vi "ProfiledPIDController_Calculate_Meas.vi"(10 "PV-Measurement":dbl, 11 "in PROFILED_PID_CONTROLLER":T1={"Controller"={"Kp"=0.0, "Ki"=0.0, "Kd"=0.0, "Period"=0.0, "Max_Integral"=1.0, "Min_Integral"=-1.0, "Max_Input"=0.0, "Min_Input"=0.0, "Continuous"=FALSE, "PositionError"=0.0, "VelocityError"=0.0, "PrevError"=0.0, "TotalError"=0.0, "PositionTolerance"=0.05, "VelocityTolerance"=9.99e+35, "SetPoint"=0.0, "Kf"=0.0, "Prev_Deriv"=0.0, "Prev_Deriv 2"=0.0, "DerivativeFilter"=FALSE, "Min_Output"=-9.99e+35, "Max_Output"=9.9e+35, "Prev_F_P"=0.0, "Prev_F_P_2"=0.0, "AntiWindupActive"=FALSE, "Measurement"=0.0}, "Goal"={"Position"=0.0, "Velocity"=0.0}, "Setpoint"={"Position"=0.0, "Velocity"=0.0}, "Constraint"={"MaxVelocity"=0.0, "MaxAcceleration"=0.0}} {"Constraint"."MaxAcceleration" format="%16_6e"; "Constraint"."MaxVelocity" format="%16_6e"; "Setpoint"."Velocity" format="%16_6e"; "Setpoint"."Position" format="%16_6e"; "Goal"."Velocity" format="%16_6e"; "Goal"."Position" format="%16_6e"; "Controller"."Measurement" format="%16_6e"; "Controller"."Prev_F_P_2" format="%16_6e"; "Controller"."Prev_F_P" format="%16_6e"; "Controller"."Max_Output" format="%16_6e"; "Controller"."Min_Output" format="%16_6e"; "Controller"."Prev_Deriv 2" format="%16_6e"; "Controller"."Prev_Deriv" format="%16_6e"; "Controller"."Kf" format="%16_6e"; "Controller"."SetPoint" format="%16_6e"; "Controller"."VelocityTolerance" format="%16_6e"; "Controller"."PositionTolerance" format="%16_6e"; "Controller"."TotalError" format="%16_6e"; "Controller"."PrevError" format="%16_6e"; "Controller"."VelocityError" format="%16_6e"; "Controller"."PositionError" format="%16_6e"; "Controller"."Min_Input" format="%16_6e"; "Controller"."Max_Input" format="%16_6e"; "Controller"."Min_Integral" format="%16_6e"; "Controller"."Max_Integral" format="%16_6e"; "Controller"."Period" format="%16_6e"; "Controller"."Kd" format="%16_6e"; "Controller"."Ki" format="%16_6e"; "Controller"."Kp" format="%16_6e"}) -> (1 "CO-ControlOutput":dbl, 3 "out PROFILED_PID_CONTROLLER":T1={"Controller"={"Kp"=0.0, "Ki"=0.0, "Kd"=0.0, "Period"=0.0, "Max_Integral"=1.0, "Min_Integral"=-1.0, "Max_Input"=0.0, "Min_Input"=0.0, "Continuous"=FALSE, "PositionError"=0.0, "VelocityError"=0.0, "PrevError"=0.0, "TotalError"=0.0, "PositionTolerance"=0.05, "VelocityTolerance"=9.99e+35, "SetPoint"=0.0, "Kf"=0.0, "Prev_Deriv"=0.0, "Prev_Deriv 2"=0.0, "DerivativeFilter"=FALSE, "Min_Output"=-9.99e+35, "Max_Output"=9.9e+35, "Prev_F_P"=0.0, "Prev_F_P_2"=0.0, "AntiWindupActive"=FALSE, "Measurement"=0.0}, "Goal"={"Position"=0.0, "Velocity"=0.0}, "Setpoint"={"Position"=0.0, "Velocity"=0.0}, "Constraint"={"MaxVelocity"=0.0, "MaxAcceleration"=0.0}} {"Constraint"."MaxAcceleration" format="%16_6e"; "Constraint"."MaxVelocity" format="%16_6e"; "Setpoint"."Velocity" format="%16_6e"; "Setpoint"."Position" format="%16_6e"; "Goal"."Velocity" format="%16_6e"; "Goal"."Position" format="%16_6e"; "Controller"."Measurement" format="%16_6e"; "Controller"."Prev_F_P_2" format="%16_6e"; "Controller"."Prev_F_P" format="%16_6e"; "Controller"."Max_Output" format="%16_6e"; "Controller"."Min_Output" format="%16_6e"; "Controller"."Prev_Deriv 2" format="%16_6e"; "Controller"."Prev_Deriv" format="%16_6e"; "Controller"."Kf" format="%16_6e"; "Controller"."SetPoint" format="%16_6e"; "Controller"."VelocityTolerance" format="%16_6e"; "Controller"."PositionTolerance" format="%16_6e"; "Controller"."TotalError" format="%16_6e"; "Controller"."PrevError" format="%16_6e"; "Controller"."VelocityError" format="%16_6e"; "Controller"."PositionError" format="%16_6e"; "Controller"."Min_Input" format="%16_6e"; "Controller"."Max_Input" format="%16_6e"; "Controller"."Min_Integral" format="%16_6e"; "Controller"."Max_Integral" format="%16_6e"; "Controller"."Period" format="%16_6e"; "Controller"."Kd" format="%16_6e"; "Controller"."Ki" format="%16_6e"; "Controller"."Kp" format="%16_6e"})   [LabVIEW 2019, in "Trajectory_Library.lvlib"]
doc: "Returns the next output of the PID controller.\n\nInputs:\n - Profiled_PID_Controller -- Profiled_PID_Controller data cluster\n - measurement -- The current measurement of the process variable.\n\nOutputs:\n - Profiled_PID_Controller -- Updated Profiled_PID_Controller data cluster\n - CO-ControlOutput -- Calculated PID output"
uses:
  Trajectory_Library.lvlib
  PROFILED_PID_CONTROLLER.ctl
  PID_CONTROLLER.ctl
  TRAPEZOID_PROFILE_STATE.ctl
  TRAPEZOID_PROFILE_CONSTRAINT.ctl
  PIDController_SetSetpoint.vi
  PIDController_Calculate_PV.vi
  TrapProfile_ShouldFlipAcceleration.vi
  TrapProfile_Direct.vi
  <vilib>/Rock Robotics/SystemInterfaces/NetworkCommunication/NetComm_UsageReport_report.vi
  PIDController_GetPeriod.vi
  TrapProfState_New.vi
  Util_LibraryGlobals.vi
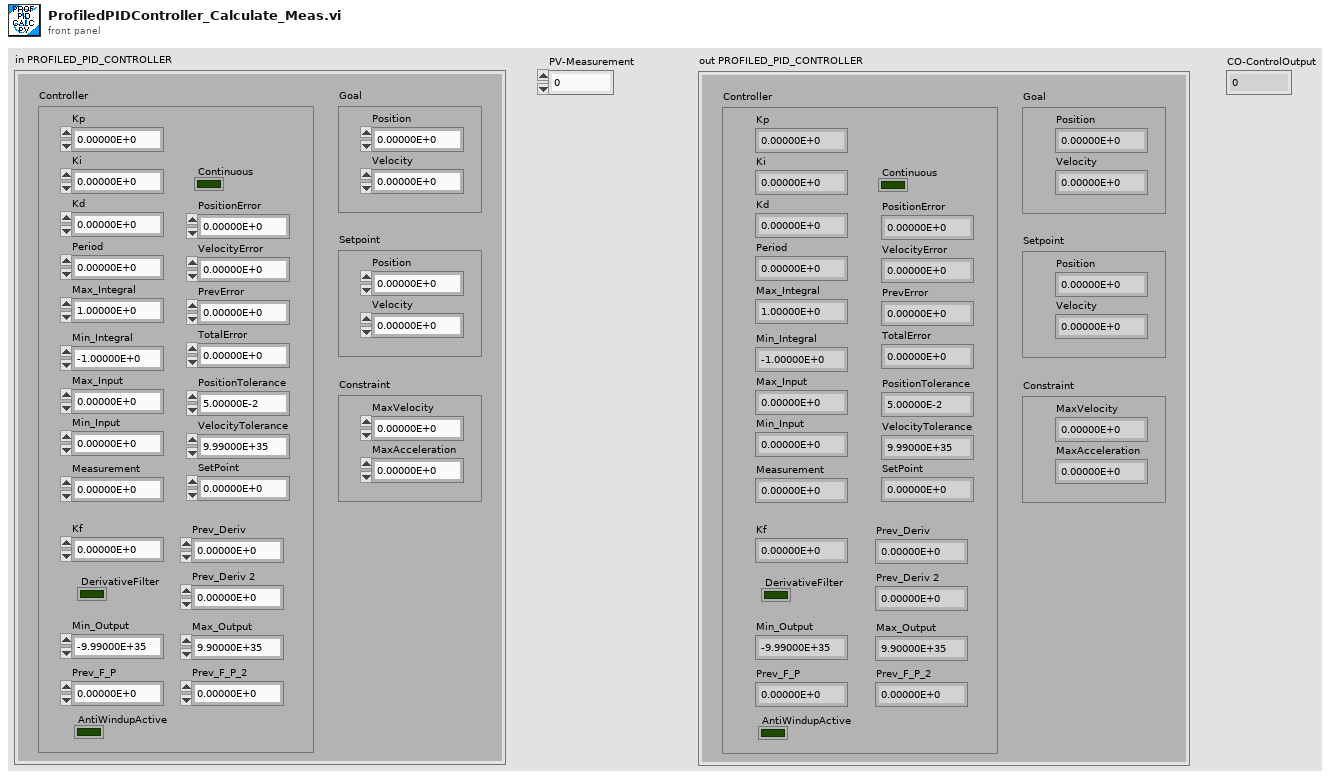
[diagram p1: front panel]
types:
  T1 = typedef "Trajectory_Library.lvlib/PROFILED_PID_CONTROLLER.ctl" = cluster{"Controller":T2, "Goal":T3, "Setpoint":T3, "Constraint":T4}
  T2 = typedef "Trajectory_Library.lvlib/PID_CONTROLLER.ctl" = cluster{"Kp":dbl, "Ki":dbl, "Kd":dbl, "Period":dbl, "Max_Integral":dbl, "Min_Integral":dbl, "Max_Input":dbl, "Min_Input":dbl, "Continuous":bool, "PositionError":dbl, "VelocityError":dbl, "PrevError":dbl, "TotalError":dbl, "PositionTolerance":dbl, "VelocityTolerance":dbl, "SetPoint":dbl, "Kf":dbl, "Prev_Deriv":dbl, "Prev_Deriv 2":dbl, "DerivativeFilter":bool, "Min_Output":dbl, "Max_Output":dbl, "Prev_F_P":dbl, "Prev_F_P_2":dbl, "AntiWindupActive":bool, "Measurement":dbl}
  T3 = typedef "Trajectory_Library.lvlib/TRAPEZOID_PROFILE_STATE.ctl" = cluster{"Position":dbl, "Velocity":dbl}
  T4 = typedef "Trajectory_Library.lvlib/TRAPEZOID_PROFILE_CONSTRAINT.ctl" = cluster{"MaxVelocity":dbl, "MaxAcceleration":dbl}
  T5 = typedef "Trajectory_Library.lvlib/TRAPEZOID_PROFILE.ctl" = cluster{"EndAccel":dbl, "EndFullSpeed":dbl, "EndDecel":dbl, "Direction":i32, "Constraints":T4, "Initial":T3, "Goal":T3}
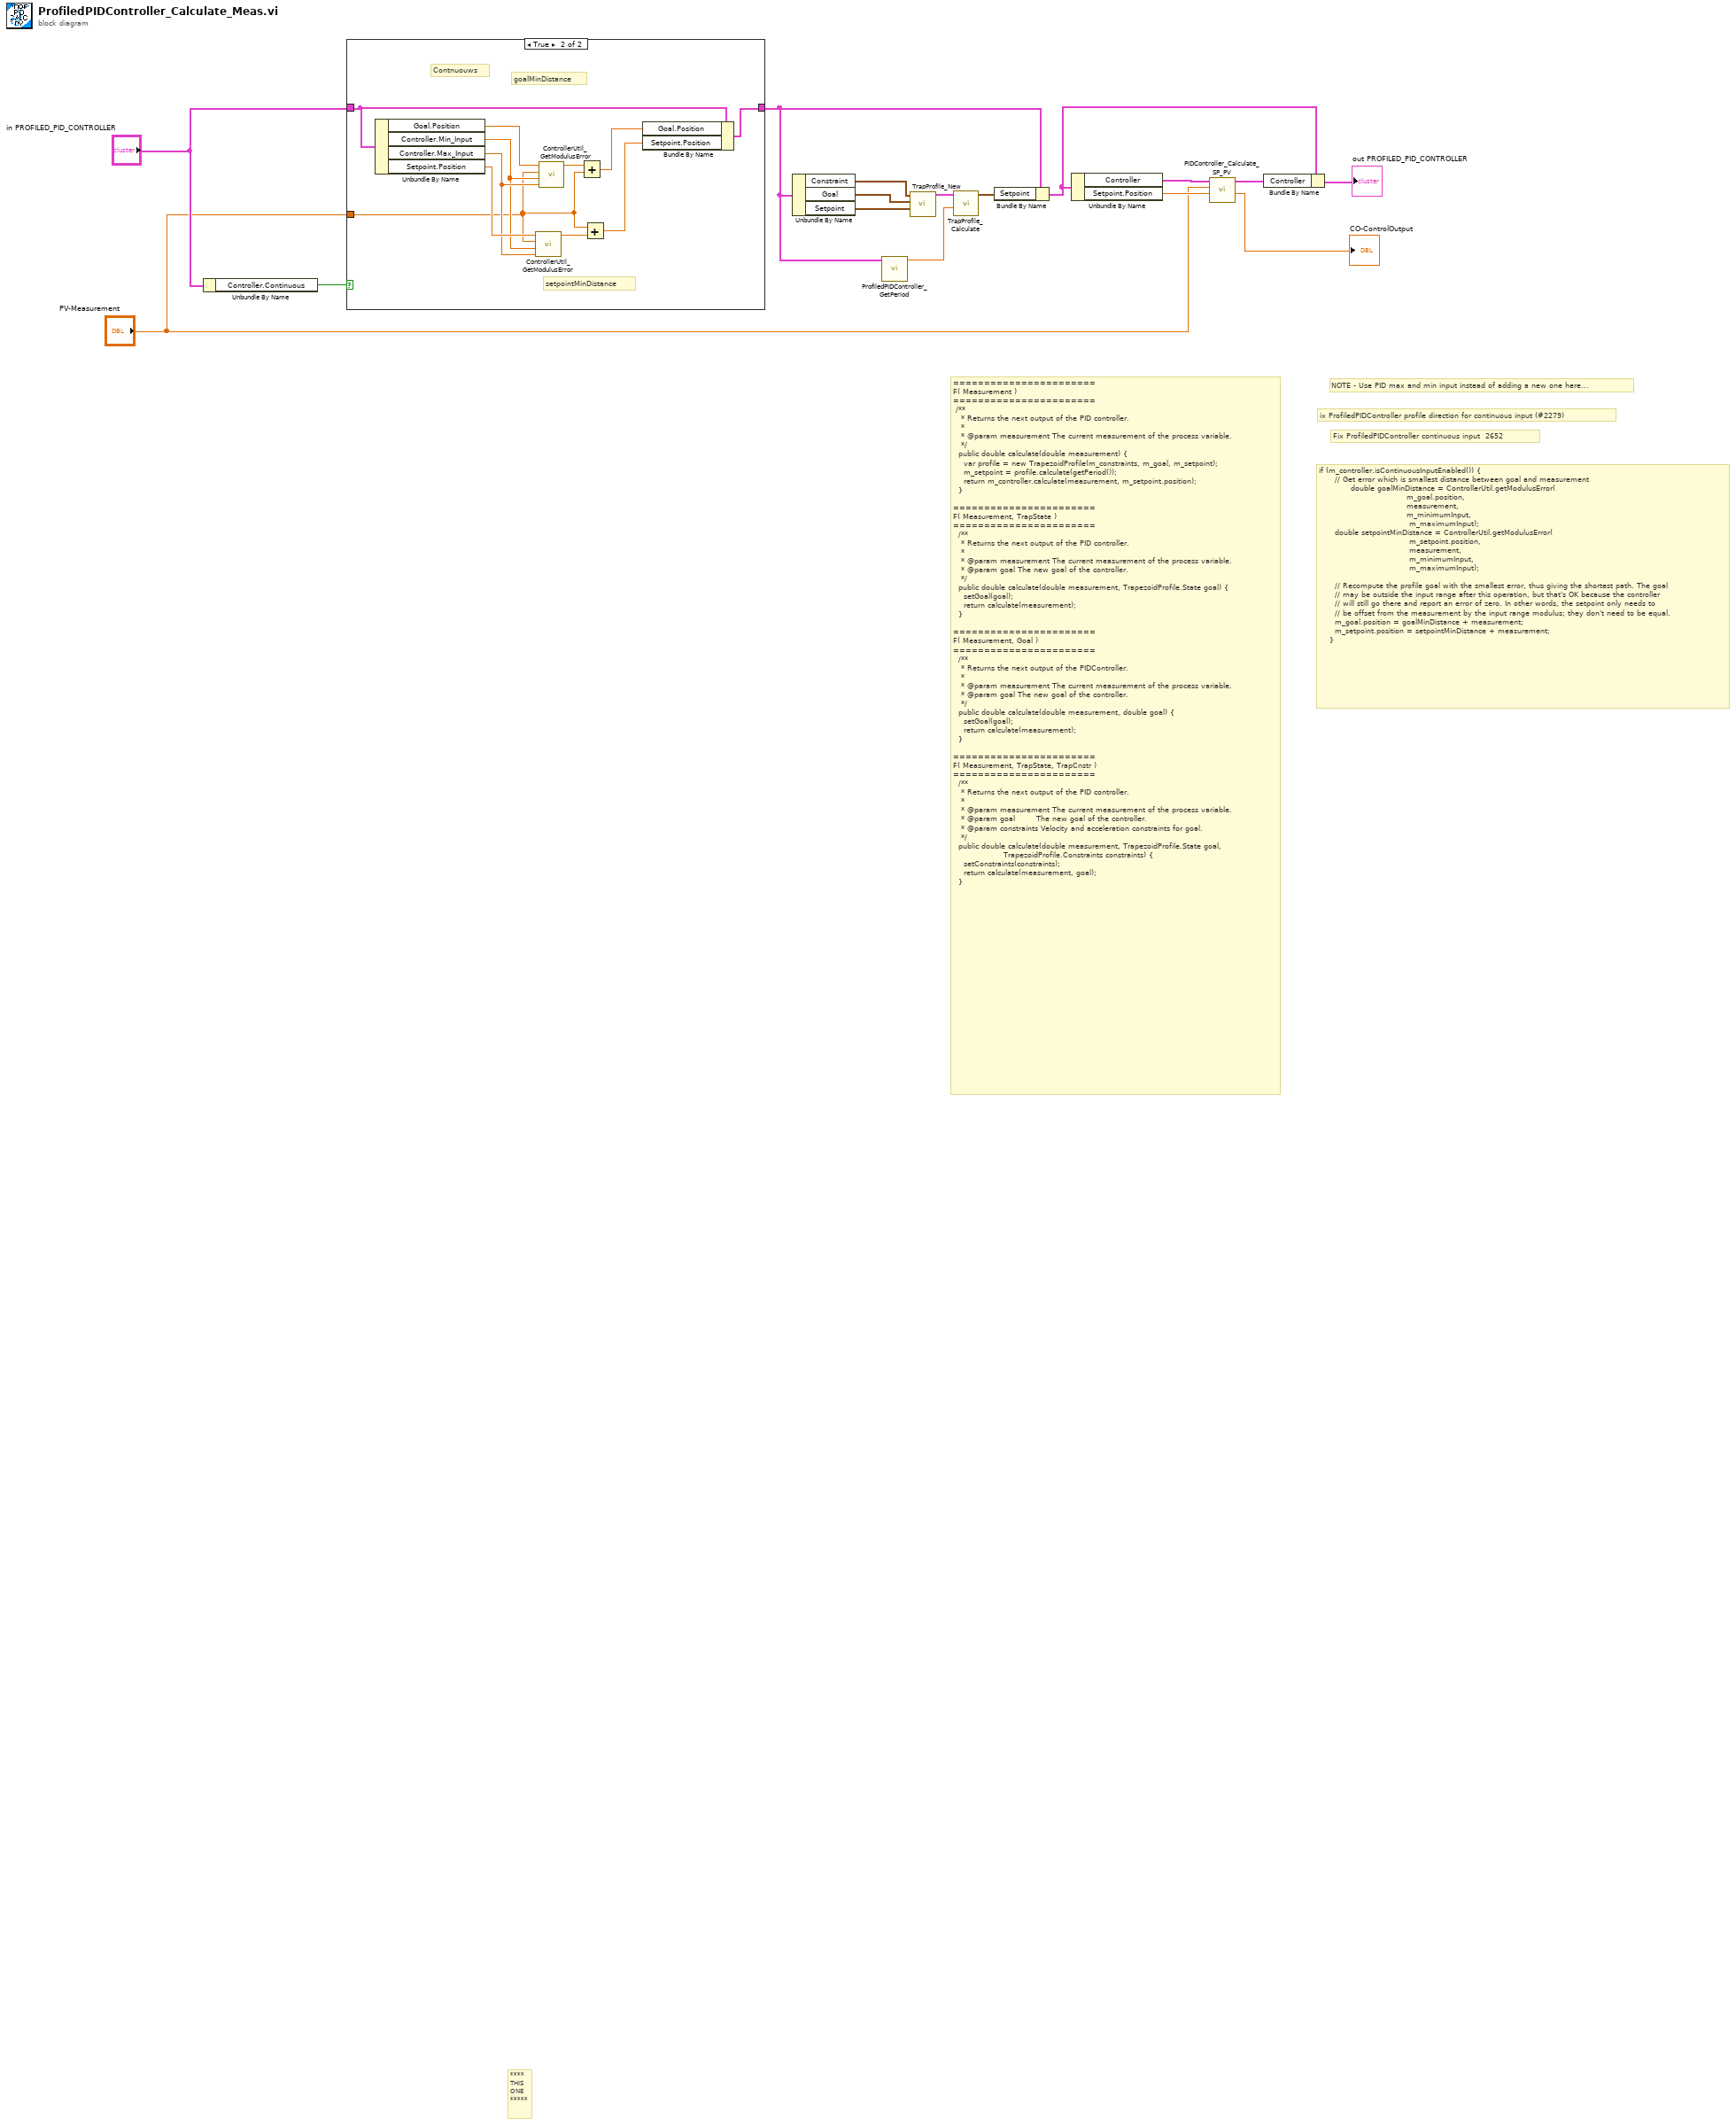
[diagram p0: block diagram]
diagram:
  # "Fix ProfiledPIDController continuous input  2652"
  # "NOTE - Use PID max and min input instead of adding a new one here..."
  # "if (m_controller.isContinuousInputEnabled()) {\n      // Get error which is smallest distance between goal and measurement\n            double goalMinDistance = ControllerUtil.getModulusError(\n                                 m_goal.position, \n                                 measurement,\n                                 m_minimumInput, \n                                  m_maximumInput);\n      double setpointMinDistance = ControllerUtil.getModulusError(\n                                  m_setpoint.position, \n                                  measurement,\n                                  m_minimumInput, \n                                  m_maximumInput);\n\n      // Recompute the profile goal with the smallest error, thus giving the shortest path. The goal\n      // may be outside the input range after this operation, but that's OK because the controller\n      // will still go there and report an error of zero. In other words, the setpoint only needs to\n      // be offset from the measurement by the input range modulus; they don't need to be equal.\n      m_goal.position = goalMinDistance + measurement;\n      m_setpoint.position = setpointMinDistance + measurement;\n    }"
  # "ix ProfiledPIDController profile direction for continuous input (#2279)"
  # "=======================\nF( Measurement ) \n=======================\n /**\n   * Returns the next output of the PID controller.\n   *\n   * @param measurement The current measurement of the process variable.\n   */\n  public double calculate(double measurement) {\n    var profile = new TrapezoidProfile(m_constraints, m_goal, m_setpoint);\n    m_setpoint = profile.calculate(getPeriod());\n    return m_controller.calculate(measurement, m_setpoint.position);\n  }\n\n=======================\nF( Measurement, TrapState ) \n=======================\n  /**\n   * Returns the next output of the PID controller.\n   *\n   * @param measurement The current measurement of the process variable.\n   * @param goal The new goal of the controller.\n   */\n  public double calculate(double measurement, TrapezoidProfile.State goal) {\n    setGoal(goal);\n    return calculate(measurement);\n  }\n\n=======================\nF( Measurement, Goal ) \n=======================\n  /**\n   * Returns the next output of the PIDController.\n   *\n   * @param measurement The current measurement of the process variable.\n   * @param goal The new goal of the controller.\n   */\n  public double calculate(double measurement, double goal) {\n    setGoal(goal);\n    return calculate(measurement);\n  }\n\n=======================\nF( Measurement, TrapState, TrapCnstr ) \n=======================\n  /**\n   * Returns the next output of the PID controller.\n   *\n   * @param measurement The current measurement of the process variable.\n   * @param goal        The new goal of the controller.\n   * @param constraints Velocity and acceleration constraints for goal.\n   */\n  public double calculate(double measurement, TrapezoidProfile.State goal,\n                   TrapezoidProfile.Constraints constraints) {\n    setConstraints(constraints);\n    return calculate(measurement, goal);\n  }"
  # "****\nTHIS\nONE\n*****"
  n1 = Unbundle By Name("in PROFILED_PID_CONTROLLER") -> ("Controller.Continuous"=w8:bool)
  n2 = case shown="True" w8 {
    tunnel: "in PROFILED_PID_CONTROLLER" -> [w17 w28]
    tunnel: [w17 w27] -> w1
    tunnel: "PV-Measurement" -> [_ w20]
    frame False {
    }
    frame True {
      # "setpointMinDistance"
      # "goalMinDistance"
      # "Contnuouws"
      n3 = Unbundle By Name(w28) -> ("Goal.Position"=w26:dbl, "Controller.Min_Input"=w21:dbl, "Controller.Max_Input"=w22:dbl, "Setpoint.Position"=w23:dbl)
      n4 = call "ControllerUtil_GetModulusError.vi"("Maximum_Input"=w22, "Minimum_Input"=w21, "Measurerment(PV)"=w20, "Reference(SP)"=w23) -> ("Error"=w18:dbl)  [unwired: 7 in]
      n5 = call "ControllerUtil_GetModulusError.vi"("Maximum_Input"=w22, "Minimum_Input"=w21, "Measurerment(PV)"=w20, "Reference(SP)"=w26) -> ("Error"=w25:dbl)  [unwired: 7 in]
      n6 = Add(x=w25, y=w20) -> (x+y=w24:dbl)
      n7 = Add(x=w20, y=w18) -> (x+y=w19:dbl)
      n8 = Bundle By Name(cluster=w28, "Goal.Position"=w24, "Setpoint.Position"=w19) -> (w27:T1)
    }
  }
  n9 = Unbundle By Name(w1) -> ("Constraint"=w3:T4, "Goal"=w5:T3, "Setpoint"=w4:T3)
  n10 = call "ProfiledPIDController_GetPeriod.vi"("in PROFILED_PID_CONTROLLER"=w1) -> ("Period"=w12:dbl)  [unwired: 10 in]
  n11 = call "TrapProfile_New.vi"("Initial"=w4, "Goal"=w5, "Constraints"=w3) -> ("TRAPEZOID_PROFILE"=w13:T5)  [unwired: 8 in]
  n12 = call "TrapProfile_Calculate.vi"("Time"=w12, "TRAPEZOID_PROFILE"=w13) -> ("State"=w11:T3)  [unwired: 9 in]
  n13 = Bundle By Name(cluster=w1, "Setpoint"=w11) -> (w10:T1)
  n14 = Unbundle By Name(w10) -> ("Controller"=w2:T2, "Setpoint.Position"=w9:dbl)
  n15 = call "PIDController_Calculate_SP_PV.vi"("SP-SetPoint"=w9, "PV-Measurement"="PV-Measurement", "in PID_CONTROLLER"=w2) -> ("CO-ControlOutput"=→"CO-ControlOutput":dbl, "out PID_CONTROLLER"=w15:T2)  [unwired: 7 in]
  n16 = Bundle By Name(cluster=w10, "Controller"=w15) -> (→"out PROFILED_PID_CONTROLLER":T1)
